vi "ShowTrainCurs.vi"(6 "Label Offset":cluster{"X":dbl, "Y":dbl}={"X"=0.0, "Y"=-40.0}, 10 "value":T1[](array[typedef]), 11 "Map":refnum<vi>) -> (3 "Map out":refnum<vi>)   [LabVIEW 2014]
uses:
  Libraries/Contact Data/Contact.ctl
  Libraries/Contact Data/Position.ctl
  Libraries/Contact Data/Controls.ctl
  Libraries/Contact Data/DestinationCluster.ctl
  Libraries/Contact Data/DesinationControls.ctl
  Libraries/Contact Data/Contact Data.lvlib
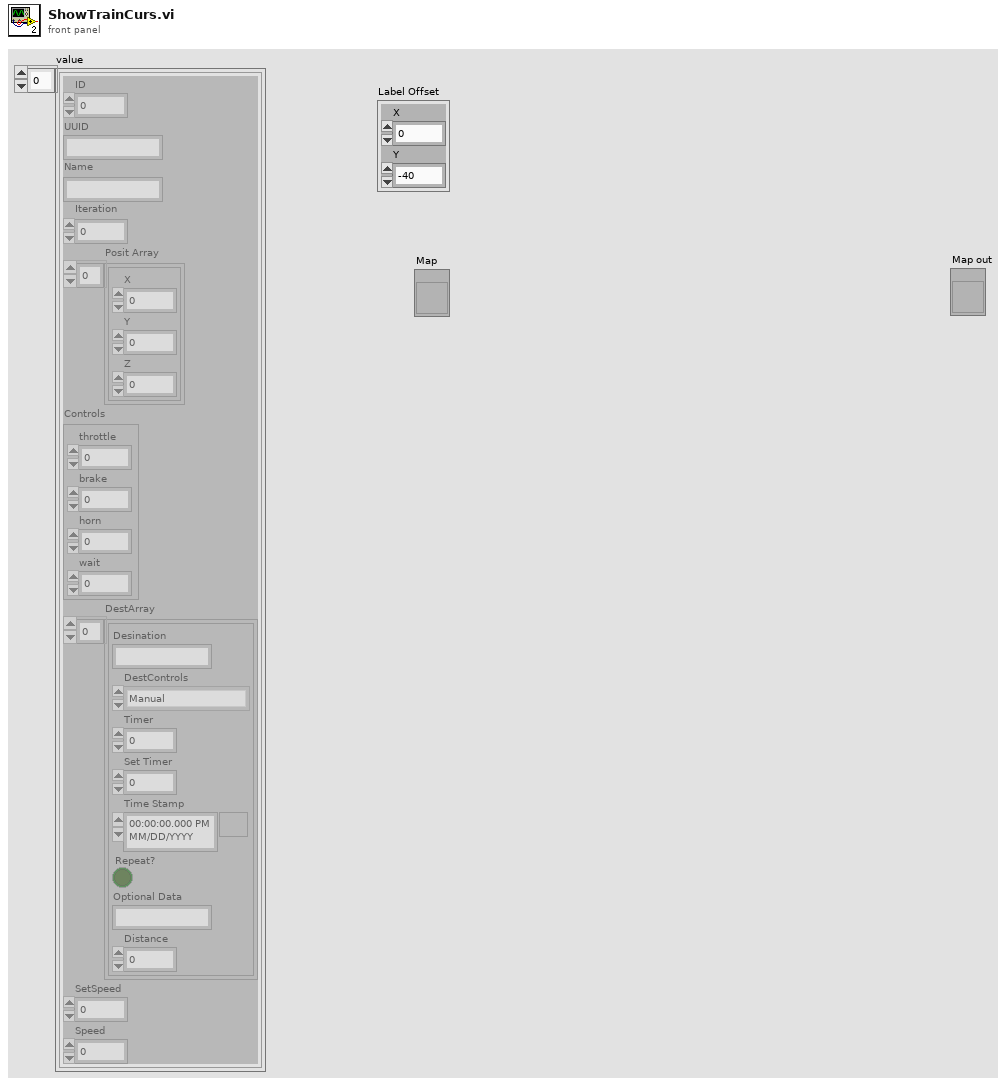
[diagram p1: front panel]
types:
  T1 = typedef "Contact Data.lvlib/Contact.ctl" = cluster{"ID":u32, "UUID":string, "Name":string, "Iteration":i32, "Posit Array":T2[], "Controls":T3, "DestArray":T4[], "SetSpeed":dbl, "Speed":dbl}
  T2 = typedef "Contact Data.lvlib/Position.ctl" = cluster{"X":dbl, "Y":dbl, "Z":dbl}
  T3 = typedef "Contact Data.lvlib/Controls.ctl" = cluster{"throttle":dbl, "brake":dbl, "horn":dbl, "wait":dbl}
  T4 = typedef "Contact Data.lvlib/DestinationCluster.ctl" = cluster{"Desination":string, "DestControls":T5, "Timer":u32, "Set Timer":u32, "Time Stamp":timestamp, "Repeat?":bool, "Optional Data":string, "Distance":dbl}
  T5 = typedef "Contact Data.lvlib/DesinationControls.ctl" = enum16{"Tracker", "Manual", "Stop", "Station DateTime", "Station Timer", "Maintain"}
  T6 = typedef "LVCursorListTypeDef.ctl" = cluster{"Name":string, "Color":u32, "Style":u8, "Point Style":u8, "Name Visible":bool, "Allow Drag":bool, "Cursor Mode":u32, "Plot":i32, "Index":i32, "Position":cluster{"X":dbl, "Y":dbl}, "X Scale":u32, "Y Scale":u32, "Watch Plots":i32[], "Watch All Plots":bool, "Plot Area":i32, "Label Offset":cluster{"X":dbl, "Y":dbl}}[]
  T7 = cluster{"Name":string, "Color":u32, "Style":u8, "Point Style":u8, "Name Visible":bool, "Allow Drag":bool, "Cursor Mode":u32, "Plot":i32, "Index":i32, "Position":cluster{"X":dbl, "Y":dbl}, "X Scale":u32, "Y Scale":u32, "Watch Plots":i32[], "Watch All Plots":bool, "Plot Area":i32, "Label Offset":cluster{"X":dbl, "Y":dbl}}
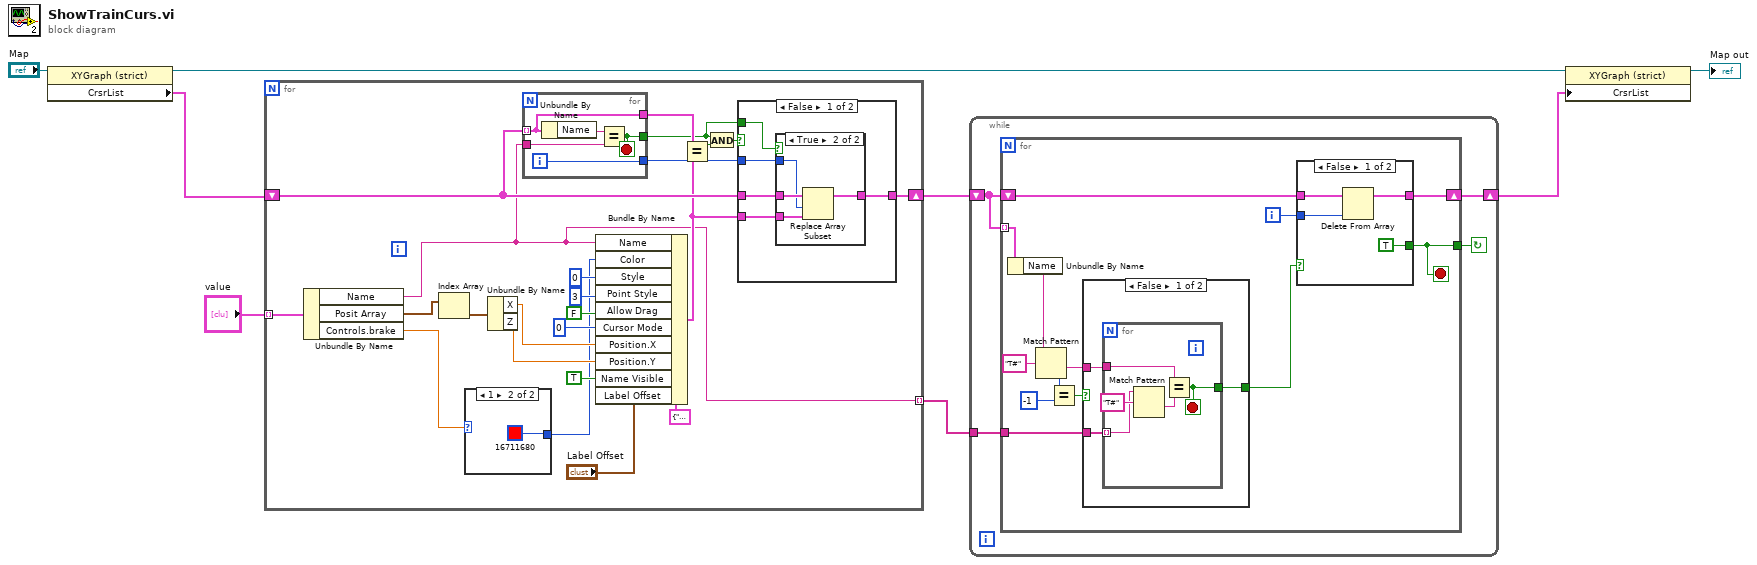
[diagram p0: block diagram]
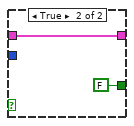
[diagram p2: hidden frame]
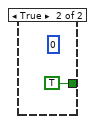
[diagram p3: hidden frame]
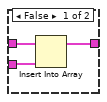
[diagram p4: hidden frame]
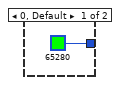
[diagram p6: hidden frame]
diagram:
  n1 = property on="Property Node" class="XYGraph (strict)"(reference="Map") -> (reference out=w6:refnum<vi>, "CrsrList"=w4:T6)  [unwired: 1 in, 1 out]
  n2 = for {
    tunnel: "value" -> [w20] mode=indexing
    shift-right: [w31] -> w2
    shift-left: w4 -> [w19]
    tunnel: [w10] -> w3 mode=indexing
    n3 = Unbundle By Name(w20) -> ("Name"=w10:string, "Posit Array"=w12:T2[], "Controls.brake"=w22:dbl)
    n4 = Index Array(array=w12) -> (element=w11:T2)  [unwired: 1 in]
    n5 = case shown="1" w22 {
      tunnel: [u32 65280 u32 16711680] -> w21
      frame 0, Default {
      }
      frame 1 {
      }
    }
    n6 = Unbundle By Name(w11) -> ("X"=w30:dbl, "Z"=w29:dbl)
    n7 = for {
      tunnel: w19 -> [w46] mode=indexing
      tunnel: w10 -> [w49]
      tunnel: [w47] -> w13
      tunnel: [w46] -> w17
      tunnel: [w45] -> w18
      i -> [w45]
      stop <- w47 stop-if-true
      n8 = Unbundle By Name(w46) -> ("Name"=w48:string)
      n9 = Equal?(x=w48, y=w49) -> (x = y?=w47:bool)
    }
    n10 = Bundle By Name(cluster=T7 {"Name"="Cursor 1", "Color"=16777222, "Style"=0, "Point Style"=6, "Name Visible"=TRUE, "Allow Drag"=TRUE, "Cursor Mode"=0, "Plot"=0, "Index"=0, "Position"={"X"=-7.216103869606, "Y"=403.5}, "X Scale"=0, "Y Scale"=0, "Watch Plots"=[], "Watch All Plots"=FALSE, "Plot Area"=0, "Label Offset"={"X"=-0.0029596755445018275, "Y"=-0.588709677419331}}, "Name"=w10, "Color"=w21, "Style"=u8 0, "Point Style"=u8 3, "Allow Drag"=FALSE, "Cursor Mode"=u32 0, "Position.X"=w30, "Position.Y"=w29, "Name Visible"=TRUE, "Label Offset"="Label Offset") -> (w16:T7)
    n11 = Equal?(x=w17, y=w16) -> (x = y?=w14:bool)
    n12 = And(x=w13, y=w14) -> (x .and. y?=w15:bool)
    n13 = case shown="False" w15 {
      tunnel: [w36 w44] -> w31
      tunnel: w16 -> [w34 _]
      tunnel: w19 -> [w35 w44]
      tunnel: w18 -> [w33 _]
      tunnel: w13 -> [w32 _]
      frame False {
        n14 = case shown="True" w32 {
          tunnel: [w38 w43] -> w36
          tunnel: w35 -> [w39 w42]
          tunnel: w34 -> [w37 w41]
          tunnel: w33 -> [_ w40]
          frame False {
            n15 = Insert Into Array(array=w39, new element=w37) -> (w38:T6)  [unwired: 1 in]
          }
          frame True {
            n16 = Replace Array Subset(array=w42, new element=w41, index=w40) -> (w43:T6)
          }
        }
      }
      frame True {
        # "no change to train"
      }
    }
  }
  n17 = while {
    tunnel: w3 -> [w55]
    shift-right: [w53] -> w1
    shift-left: w2 -> [w54]
    stop <- w52 continue-if-true
    n18 = for {
      tunnel: w55 -> [w67]
      tunnel: w54 -> [w61] mode=indexing
      shift-right: [w60] -> w53
      shift-left: w54 -> [w59]
      tunnel: [w56] -> w52
      i -> [w57]
      stop <- w56 stop-if-true
      n19 = Unbundle By Name(w61) -> ("Name"=w65:string)
      n20 = Match Pattern(string=w65, regular expression="T#") -> (after substring=w66:string, offset past match=w64:i32)  [unwired: 1 in, 2 out]
      n21 = Equal?(x=w64, y=-1) -> (x = y?=w62:bool)
      n22 = case shown="False" w62 {
        tunnel: w67 -> [w77 _]
        tunnel: w66 -> [w76 _]
        tunnel: [w75 TRUE] -> w58
        frame False {
          n23 = for {
            tunnel: w77 -> [w81] mode=indexing
            tunnel: w76 -> [w79]
            tunnel: [w78] -> w75
            stop <- w78 stop-if-true
            n24 = Match Pattern(string=w81, regular expression="T#") -> (after substring=w80:string)  [unwired: 1 in, 3 out]
            n25 = Equal?(x=w79, y=w80) -> (x = y?=w78:bool)
          }
        }
        frame True {
          (unwired) 0
        }
      }
      n26 = case shown="False" w58 {
        tunnel: w59 -> [w72 w74]
        tunnel: [w71 w74] -> w60
        tunnel: w57 -> [w70 _]
        tunnel: [TRUE FALSE] -> w56
        frame False {
          n27 = Delete From Array(array=w72, index=w70) -> (array with subset deleted=w71:T6)  [unwired: 1 in, 1 out]
        }
        frame True {
        }
      }
    }
  }
  n28 = property on="Property Node" class="XYGraph (strict)"(reference=w6, "CrsrList"=w1) -> (reference out=→"Map out":refnum<vi>)  [unwired: 1 in, 1 out]
